vi "Write String.vi"(8 "error in (no error)":errorcluster, 9 "offset (0)":i64, 10 "string in":string, 11 "pointer in":u64) -> (0 "error out":errorcluster, 1 "offset out":i64, 2 "bytes written":i64, 3 "pointer out":u64)   [LabVIEW 2013, in "Linux RT IPC.lvlib" / "Shared Memory.lvlib"]
uses:
  Shared Memory.lvlib
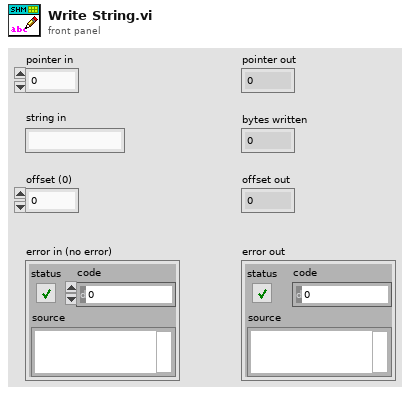
[diagram p1: front panel]
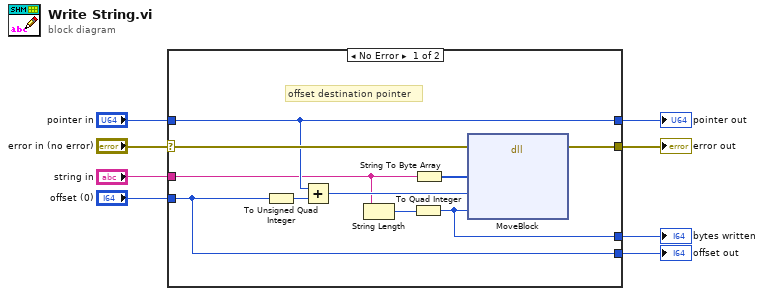
[diagram p0: block diagram]
diagram:
  n1 = case shown="No Error" "error in (no error)" {
    selector: "error in (no error)" -> [w17 w21]
    tunnel: [w16 w21] -> w8
    tunnel: "pointer in" -> [w14 w20]
    tunnel: "string in" -> [w11 _]
    tunnel: [w14 w20] -> w5
    tunnel: [w9 _] -> w4
    tunnel: "offset (0)" -> [w13 w19]
    tunnel: [w13 w19] -> w2
    frame No Error {
      # "offset destination pointer"
      n2 = To Unsigned Quad Integer(1:w13) -> (0:w18:u64)
      n3 = Add(x=w14, y=w18) -> (x+y=w15:u64)
      n4 = String Length(string=w11) -> (length=w10:i32)
      n5 = To Quad Integer(1:w10) -> (0:w9:i64)
      n6 = String To Byte Array(string=w11) -> (unsigned byte array=w12:u8[])
      n7 = dll-call lib="LabVIEW" fn="MoveBlock"(error in=w17, "data"=w12, "pointer"=w15, "size"=w9) -> (error out=w16:errorcluster)  [unwired: 6 in, 1 out]
    }
    frame Error {
    }
  }
  "error out" <- w8
  "pointer out" <- w5
  "bytes written" <- w4
  "offset out" <- w2
